vi "cm2nm_create_list_of_spots.vi"(0 "Current Session":T1) -> (1 "Indices_Experimental_positions":i32[](array[numeric]), 2 "Indices of calculated positions":i32[](array[numeric]), 3 "labels_Experimental_positions":string[](array[string]), 4 "Name of calculated positions":string[](array[string]))   [LabVIEW 2011]
doc: "Loop through the current session spots (collection of points) to create a list of spots that have \"experimental\" values and those that have been calculated from previous sessions. Lists are made of the names and the indices from the current session spot array. The list of names are needed to supply drop down lists in the GUI."
uses:
  cm2nm_sample_set.ctl
  cm2nm_coordinate_information_v2.ctl
  Instrument_type_enum_v2.ctl
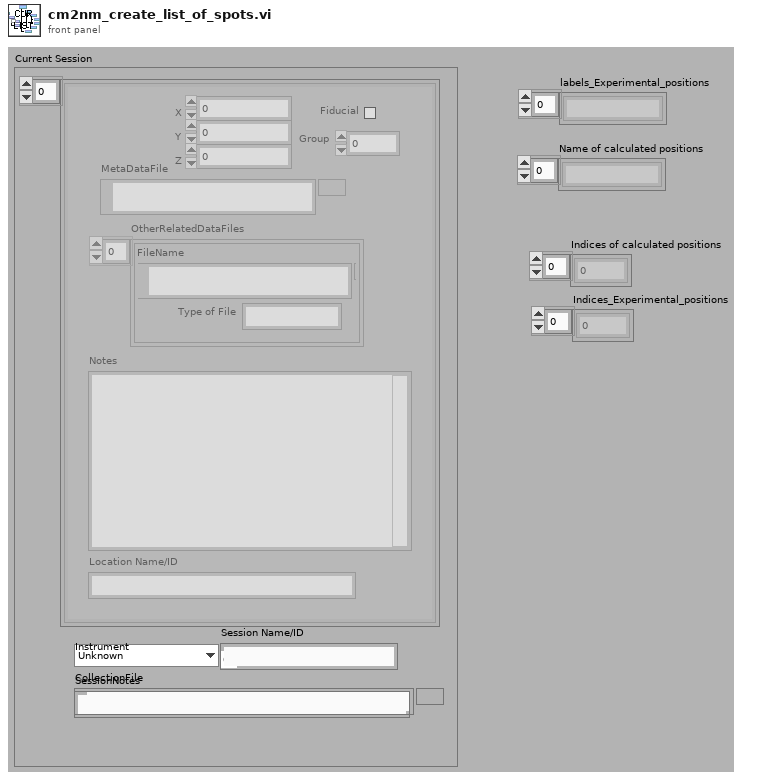
[diagram p1: front panel]
types:
  T1 = typedef "cm2nm_sample_set.ctl" = cluster{"CollectionOfPoints":T2[], "Instrument":T3, "CollectionFile":path, "Session Name/ID":string, "SessionNotes":string}
  T2 = typedef "cm2nm_coordinate_information_v2.ctl" = cluster{"MetaDataFile":path, "X":dbl, "Y":dbl, "Z":dbl, "Group":i32, "Rotation":dbl[unit], "Fiducial":bool, "Magnification":dbl, "Working_Distance":dbl, "Notes":string, "Location Name/ID":string, "OtherRelatedDataFiles":cluster{"Type of File":string, "FileName":path}[], "Available":bool}
  T3 = typedef "Instrument_type_enum_v2.ctl" = enum16{"Unknown", "Philips FEI SEM IRC", "JEOL 7000F EML_MFC", "MXRD MFC", "JEOL_EPMA"}
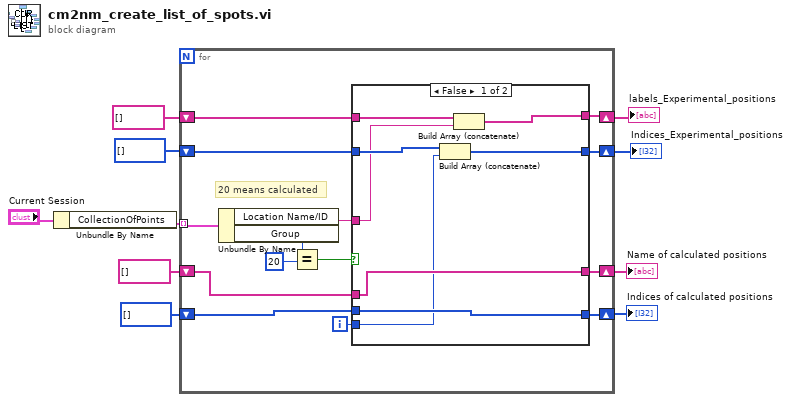
[diagram p0: block diagram]
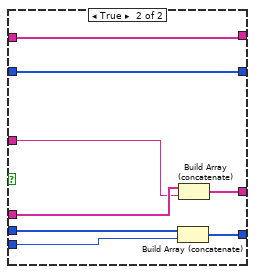
[diagram p2: hidden frame]
diagram:
  n1 = Unbundle By Name("Current Session") -> ("CollectionOfPoints"=w5:T2[])
  n2 = for {
    tunnel: w5 -> [w21] mode=indexing
    shift-right: [w19] -> w8
    shift-left: string[] [] -> [w18]
    shift-right: [w17] -> w9
    shift-left: i32[] [] -> [w16]
    shift-right: [w11] -> w2
    shift-left: string[] [] -> [w12]
    shift-right: [w13] -> w1
    shift-left: i32[] [] -> [w14]
    i -> [w20]
    # "20 means calculated"
    n3 = Unbundle By Name(w21) -> ("Location Name/ID"=w15:string, "Group"=w24:i32)
    n4 = Equal?(x=w24, y=20) -> (x = y?=w22:bool)
    n5 = case shown="False" w22 {
      tunnel: w20 -> [w29 w38]
      tunnel: [w32 w40] -> w19
      tunnel: w18 -> [w32 w39]
      tunnel: [w31 w37] -> w17
      tunnel: w16 -> [w31 w36]
      tunnel: w15 -> [w25 w35]
      tunnel: w14 -> [w30 w34]
      tunnel: [w28 w34] -> w13
      tunnel: w12 -> [w27 w33]
      tunnel: [w26 w33] -> w11
      frame False {
        n6 = Build Array (concatenate)(w30, w29) -> (w28:i32[])
        n7 = Build Array (concatenate)(w27, w25) -> (w26:string[])
      }
      frame True {
        n8 = Build Array (concatenate)(w36, w38) -> (w37:i32[])
        n9 = Build Array (concatenate)(w39, w35) -> (w40:string[])
      }
    }
  }
  "Indices of calculated positions" <- w9
  "Name of calculated positions" <- w8
  "labels_Experimental_positions" <- w2
  "Indices_Experimental_positions" <- w1
